vi "st_Binomial CDF (kx).vi"(9 "a":dbl=0.02, 10 "n":i32=100, 11 "x":dbl) -> (0 "error":i32, 3 "cdf(x)":dbl=0.13261955589475294)   [LabVIEW 2020, in "NI_Gmath.lvlib"]
doc: "Computes the one-sided <B>probability</B>, p, of the normally distributed random variable, <B>x</B>."
uses:
  <vilib>/gmath/NI_Gmath.lvlib
  <vilib>/gmath/statdist.llb/st_error_code.ctl
  <vilib>/gmath/SpecialFunctions.llb/Incomplete Beta Function.vi
panel:
  # "Binomial CDF"
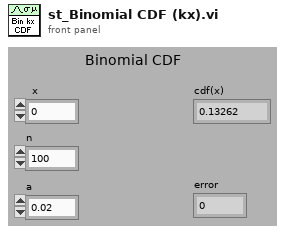
[diagram p1: front panel]
types:
  T1 = typedef "NI_Gmath.lvlib/st_error_code.ctl" = i32
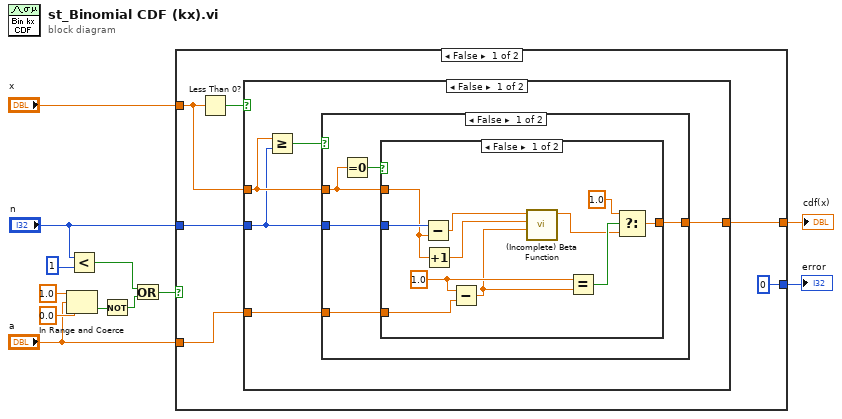
[diagram p0: block diagram]
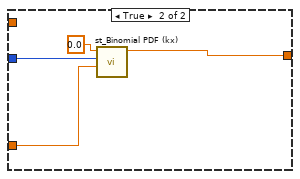
[diagram p2: hidden frame]
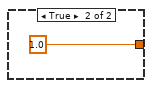
[diagram p3: hidden frame]
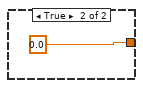
[diagram p4: hidden frame]
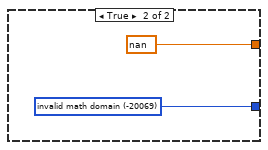
[diagram p5: hidden frame]
diagram:
  n1 = In Range and Coerce(upper limit=1.0, x="a", lower limit=0.0) -> (In Range?=w4:bool)  [unwired: 1 out]
  n2 = Less?(x="n", y=1) -> (x < y?=w2:bool)
  n3 = Not(x=w4) -> (.not. x?=w3:bool)
  n4 = Or(x=w2, y=w3) -> (x .or. y?=w7:bool)
  n5 = case shown="False" w7 {
    tunnel: [0 ("invalid math domain") w46] -> w12
    tunnel: [w17 nan] -> w11
    tunnel: "x" -> [w13 _]
    tunnel: "n" -> [w16 _]
    tunnel: "a" -> [w15 _]
    frame False {
      n6 = Less Than 0?(x=w13) -> (x < 0?=w14:bool)
      n7 = case shown="False" w14 {
        tunnel: [w22 0.0] -> w17
        tunnel: w13 -> [w21 _]
        tunnel: w16 -> [w20 _]
        tunnel: w15 -> [w19 _]
        frame False {
          n8 = Greater Or Equal?(x=w21, y=w20) -> (x >= y?=w23:bool)
          n9 = case shown="False" w23 {
            tunnel: [w25 1.0] -> w22
            tunnel: w21 -> [w24 _]
            tunnel: w20 -> [w27 _]
            tunnel: w19 -> [w26 _]
            frame False {
              n10 = Equal To 0?(x=w24) -> (x = 0?=w28:bool)
              n11 = case shown="False" w28 {
                tunnel: w27 -> [w39 w41]
                tunnel: w26 -> [w37 w42]
                tunnel: [w33 w40] -> w25
                tunnel: w24 -> [w38 _]
                frame False {
                  w36 = 1.0
                  n12 = Subtract(x=w39, y=w38) -> (x-y=w32:dbl)
                  n13 = Increment(x=w38) -> (x+1=w31:dbl)
                  n14 = Subtract(x=w36, y=w37) -> (x-y=w30:dbl)
                  n15 = call-poly <vilib>:"(Incomplete) Beta Function.vi"("a"=w30, "y"=w31, "x"=w32) -> ("b(x, y, a)"=w29:dbl)  [unwired: 8 in]
                  n16 = Equal?(x=w36, y=w30) -> (x = y?=w34:bool)
                  n17 = Select(t=1.0, s=w34, f=w29) -> (s? t:f=w33:dbl)
                }
                frame True {
                  n18 = call <vilib>:"st_Binomial PDF (kx).vi"("p"=w42, "n"=w41, "x"=0.0 ("a")) -> ("pdf(x)"=w40:dbl)  [unwired: 7 in, 1 out]
                }
              }
            }
            frame True {
            }
          }
        }
        frame True {
        }
      }
    }
    frame True {
      w46 = T1 -20069 items=["invalid math domain"=-20069, "Fourier interpolation size m >= n"=-20070, "empty array"=-20003] ("stat interp error code")
    }
  }
  "cdf(x)" <- w11
  "error" <- w12
